vi "IMAQdx Calculate Frames per Second 1.vi"(0 "Session In":T1, 5 "Buffer Number":u32, 7 "Minimum Display Update Interval (ms)":u32=1000, 9 "Frames per Second Update Interval (ms)":u32=1000, 11 "error in (no error)":errorcluster, 12 "Reset Counters":bool) -> (3 "Update Display":bool, 4 "Session Out":T1, 6 "Acquired Frames per Second":dbl, 8 "Processed Frames per Second":dbl, 10 "Images Behind":i32, 14 "Images Missed":u32, 15 "error out":errorcluster)   [LabVIEW 2025, in "NI_Vision_Acquisition_Software.lvlib"]
doc: "Calculates the acquired and processing frame rate, the images behind, and images missed. This VI operates on a per-session basis, so it can be called with different IMAQdx camera sessions in parallel and it will return the calculated values for the session passed in."
uses:
  <vilib>/vision/driver/NI_Vision_Acquisition_Software.lvlib
  <vilib>/userDefined/High Color/IMAQdx.ctl
  <resource>/objmgr/imaqdx.rc
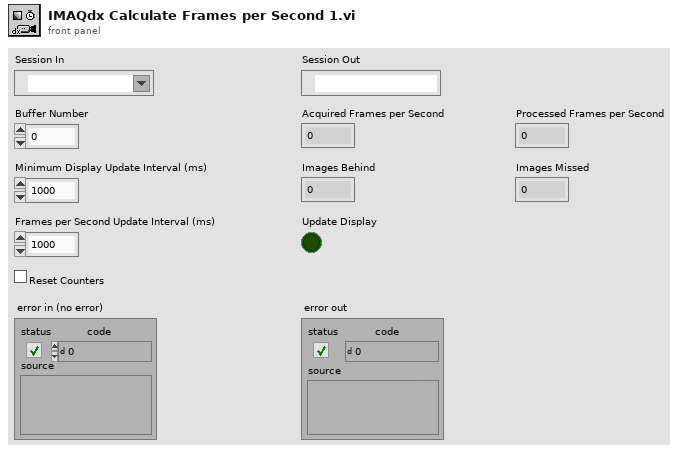
[diagram p1: front panel]
types:
  T1 = typedef "IMAQdx.ctl" = refnum<k21>
  T2 = cluster{"Last Display Timer Value":u32, "Last FPS Timer Value":u32, "Previous Buffer Number":i32, "Images Missed":u32, "Total Camera Frames":i32, "Last Acquired Frame Rate":dbl, "Last Processed Frame Rate":dbl, "Last Number of Processed Images":u32}
  T3 = cluster{"Last Display Timer Value":u32, "Last FPS Timer Value":u32, "Previous Buffer Number":i32, "Images Missed":u32, "Total Camera Frames":i32, "Last Acquired Frame Rate":dbl, "Last Processed Frame Rate":dbl, "Last Number of Processed Images":u32}[]
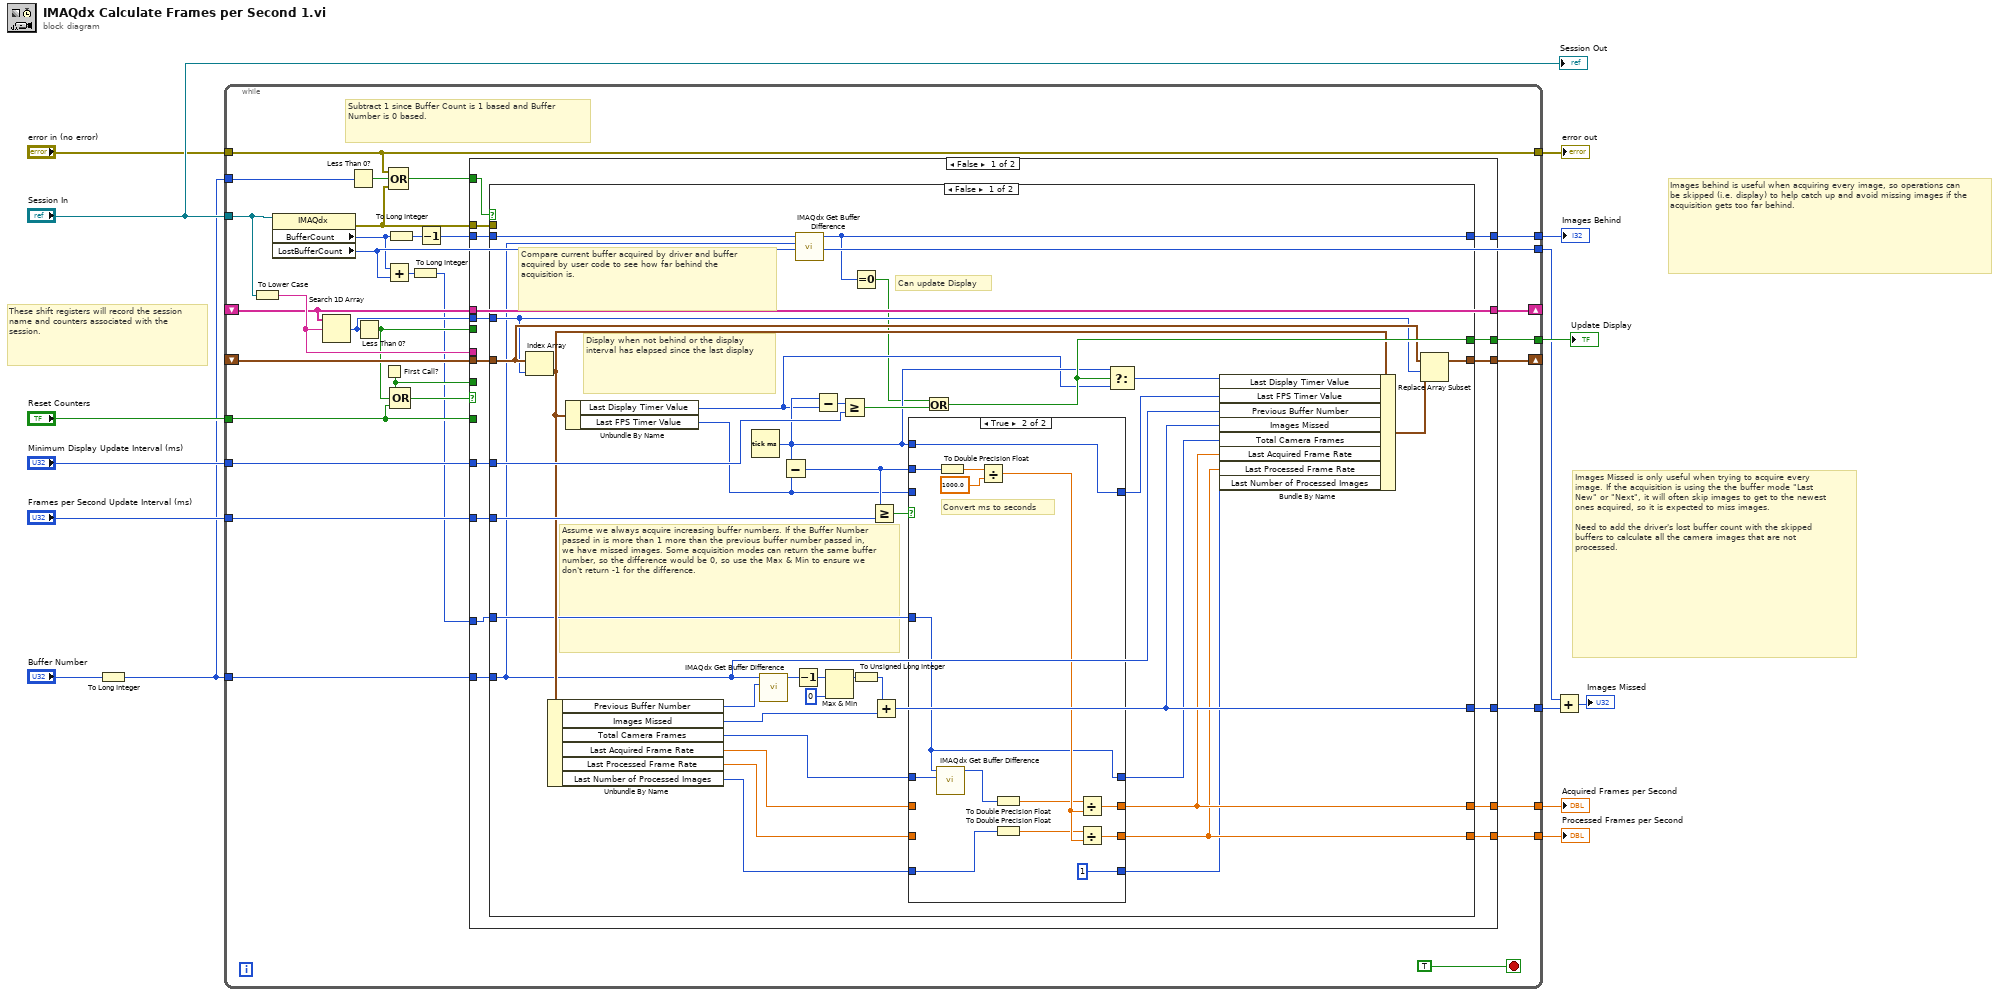
[diagram p0: block diagram]
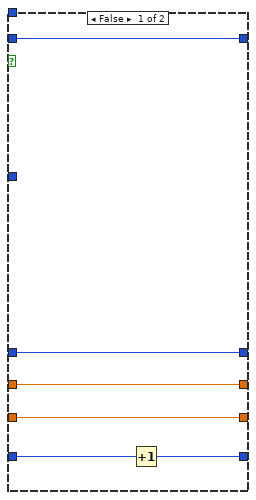
[diagram p2: hidden frame]
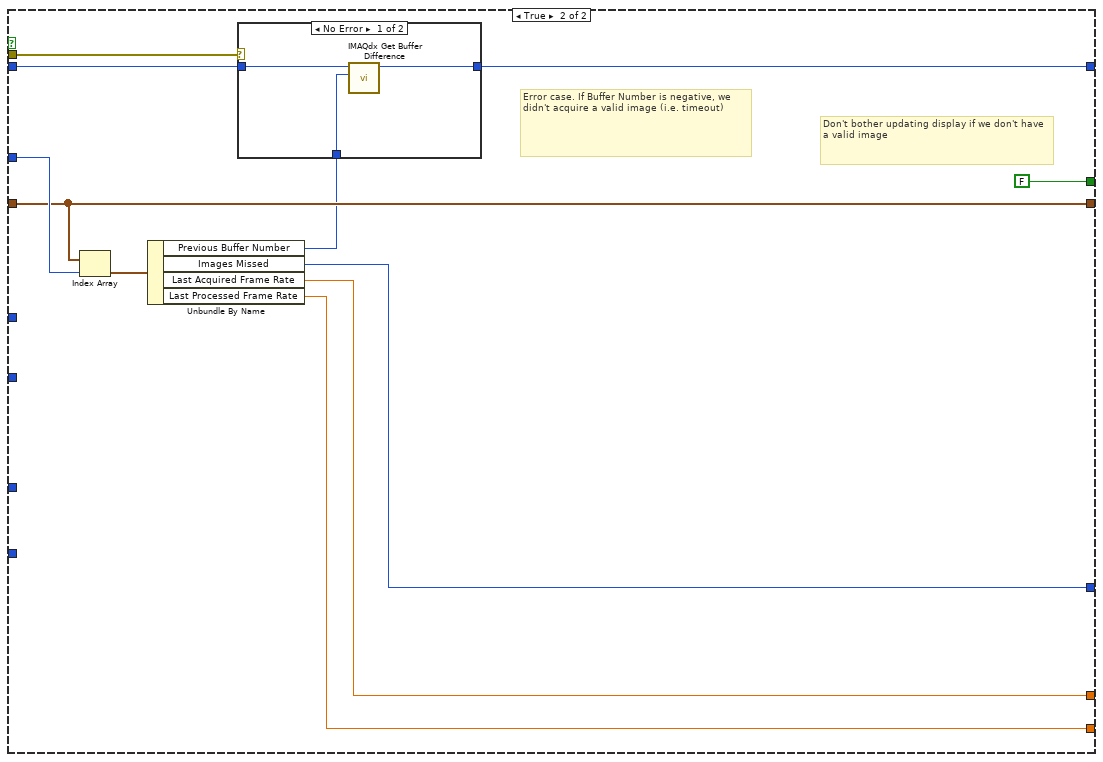
[diagram p3: hidden frame]
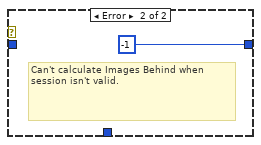
[diagram p4: hidden frame]
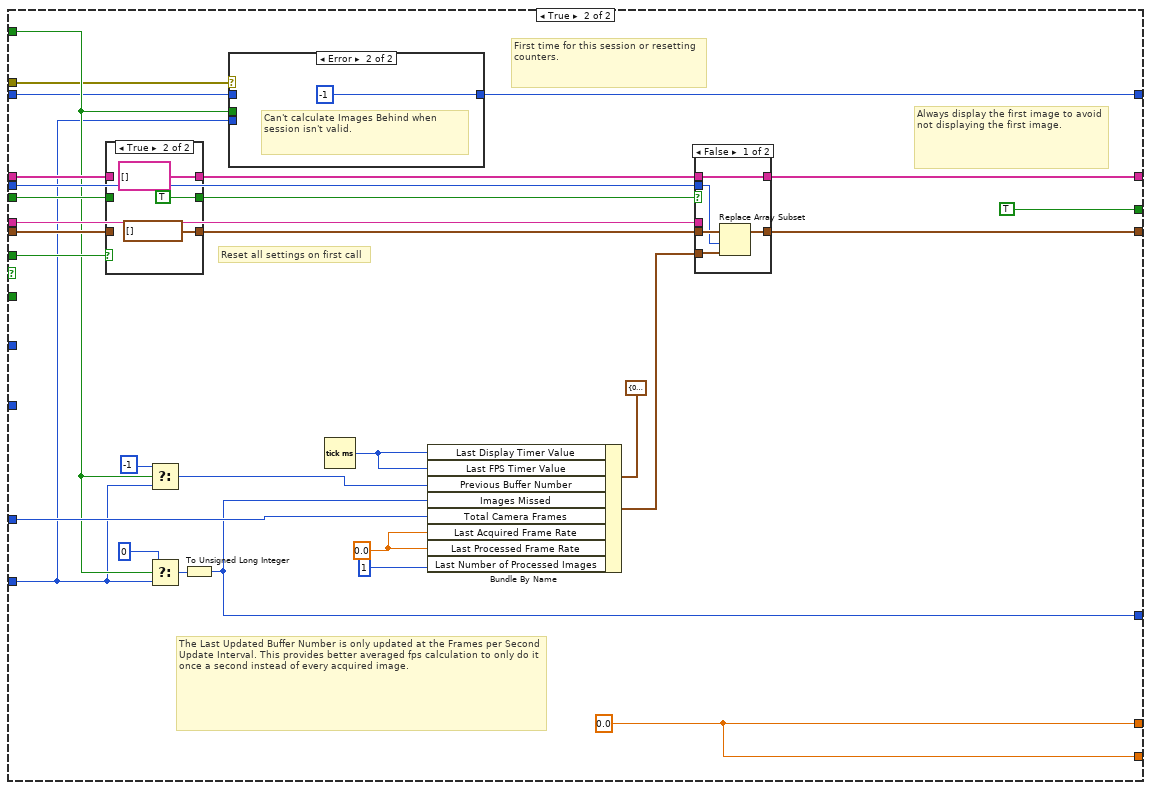
[diagram p5: hidden frame]
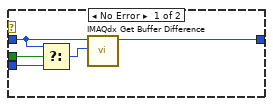
[diagram p6: hidden frame]
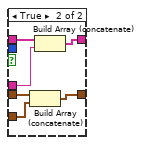
[diagram p8: hidden frame]
diagram:
  # "These shift registers will record the session name and counters associated with the session."
  # "Images behind is useful when acquiring every image, so operations can be skipped (i.e. display) to help catch up and avoid missing images if the acquisition gets too far behind."
  # "Images Missed is only useful when trying to acquire every image. If the acquisition is using the the buffer mode \"Last New\" or \"Next\", it will often skip images to get to the newest ones acquired, so it is expected to miss images. \n\nNeed to add the driver's lost buffer count with the skipped buffers to calculate all the camera images that are not processed."
  n1 = To Long Integer(number="Buffer Number") -> (32bit integer=w1:i32)
  n2 = while {
    tunnel: "Minimum Display Update Interval (ms)" -> [w45]
    tunnel: w1 -> [w44]
    tunnel: "Reset Counters" -> [w31]
    tunnel: "Session In" -> [w28]
    tunnel: [w19] -> w12
    tunnel: [w43] -> w11
    tunnel: "Frames per Second Update Interval (ms)" -> [w42]
    tunnel: [w24] -> w9
    tunnel: "error in (no error)" -> [w24]
    shift-right: [w41] -> _
    shift-left: _ -> [w40]
    tunnel: [w39] -> w5
    tunnel: [w38] -> w7
    tunnel: [w37] -> w6
    shift-right: [w34] -> _
    shift-left: _ -> [w33]
    tunnel: [w26] -> w4
    tunnel: w1 -> [w22]
    stop <- TRUE stop-if-true
    # "Subtract 1 since Buffer Count is 1 based and Buffer Number is 0 based."
    n3 = To Lower Case(string=w28) -> (all lower case string=w35:string)
    n4 = property class="IMAQdx"(reference=w28) -> (error out=w16:errorcluster, "BufferCount"=w20:u32, "LostBufferCount"=w26:u32)  [unwired: 1 in, 1 out]
    n5 = Search 1D Array(1D array=w33, element=w35) -> (index of element=w32:i32)  [unwired: 1 in]
    n6 = Less Than 0?(x=w22) -> (x < 0?=w25:bool)
    n7 = Less Than 0?(x=w32) -> (x < 0?=w30:bool)
    n8 = First Call?() -> (First Call?: T/F=w29:bool)
    n9 = Add(x=w20, y=w26) -> (x+y=w27:u32)
    n10 = To Long Integer(number=w20) -> (32bit integer=w18:i32)
    n11 = Compound Arithmetic op=OR(w24, w25, w16) -> (w23:bool)
    n12 = Compound Arithmetic op=OR(w29, w30, w31) -> (w36:bool)
    n13 = To Long Integer(number=w27) -> (32bit integer=w21:i32)
    n14 = Decrement(x=w18) -> (x-1=w17:i32)
    n15 = case shown="False" w36 {
      tunnel: [w57 w164] -> w38
      tunnel: w44 -> [w59 w139]
      tunnel: [w56 w164] -> w37
      tunnel: [w58 w141] -> w39
      tunnel: w31 -> [_ _]
      tunnel: [w61 TRUE] -> w43
      tunnel: w45 -> [w62 _]
      tunnel: w42 -> [w60 _]
      tunnel: [w54 w157] -> w41
      tunnel: w40 -> [w53 w153]
      tunnel: w30 -> [_ w148]
      tunnel: w33 -> [w55 w151]
      tunnel: w35 -> [_ w156]
      tunnel: [w55 w155] -> w34
      tunnel: w32 -> [w52 w149]
      tunnel: w29 -> [_ w154]
      tunnel: w21 -> [w51 w146]
      tunnel: w23 -> [w50 w140]
      tunnel: w17 -> [w49 w137]
      tunnel: [w48 w138] -> w19
      tunnel: w16 -> [w47 w136]
      frame False {
        n16 = case shown="False" w50 {
          tunnel: w62 -> [w98 _]
          tunnel: [w96 FALSE] -> w61
          tunnel: w60 -> [w89 _]
          tunnel: w59 -> [w63 _]
          tunnel: [w84 w127] -> w58
          tunnel: [w75 w129] -> w57
          tunnel: [w74 w128] -> w56
          tunnel: [w70 w130] -> w54
          tunnel: w53 -> [w69 w130]
          tunnel: w52 -> [w68 w131]
          tunnel: w51 -> [w67 _]
          tunnel: w49 -> [w65 w123]
          tunnel: [w64 w126] -> w48
          tunnel: w47 -> [_ w121]
          frame False {
            # "Compare current buffer acquired by driver and buffer acquired by user code to see how far behind the acquisition is."
            # "Can update Display"
            # "Display when not behind or the display interval has elapsed since the last display"
            # "Assume we always acquire increasing buffer numbers. If the Buffer Number passed in is more than 1 more than the previous buffer number passed in, we have missed images. Some acquisition modes can return the same buffer number, so the difference would be 0, so use the Max & Min to ensure we don't return -1 for the difference."
            n17 = Index Array(array=w69, index=w68) -> (element=w83:T2)
            n18 = Unbundle By Name(w83) -> ("Previous Buffer Number"=w82:i32, "Images Missed"=w80:u32, "Total Camera Frames"=w81:i32, "Last Acquired Frame Rate"=w78:dbl, "Last Processed Frame Rate"=w77:dbl, "Last Number of Processed Images"=w73:u32)
            n19 = Unbundle By Name(w83) -> ("Last Display Timer Value"=w88:u32, "Last FPS Timer Value"=w86:u32)
            n20 = Tick Count (ms)() -> (millisecond timer value=w95:u32)
            n21 = call <vilib>:"IMAQdx Get Buffer Difference.vi"("Previous Buffer Number"=w82, "Current BufferNumber"=w63) -> ("Buffer Difference"=w93:i32)  [unwired: 9 in]
            n22 = Subtract(x=w95, y=w86) -> (x-y=w99:u32)
            n23 = Decrement(x=w93) -> (x-1=w92:i32)
            n24 = call <vilib>:"IMAQdx Get Buffer Difference.vi"("Previous Buffer Number"=w63, "Current BufferNumber"=w65) -> ("Buffer Difference"=w64:i32)  [unwired: 9 in]
            n25 = Subtract(x=w95, y=w88) -> (x-y=w94:u32)
            n26 = Max & Min(x=w92, y=0) -> (max(x,y)=w90:i32)  [unwired: 1 out]
            n27 = Greater Or Equal?(x=w94, y=w98) -> (x >= y?=w97:bool)
            n28 = Equal To 0?(x=w64) -> (x = 0?=w66:bool)
            n29 = To Unsigned Long Integer(number=w90) -> (unsigned 32bit integer=w79:u32)
            n30 = Greater Or Equal?(x=w99, y=w89) -> (x >= y?=w100:bool)
            n31 = Add(x=w79, y=w80) -> (x+y=w84:u32)
            n32 = case shown="True" w100 {
              tunnel: w86 -> [w106 _]
              tunnel: [w106 w120] -> w85
              tunnel: w81 -> [w104 w115]
              tunnel: [w104 w108] -> w76
              tunnel: w95 -> [_ w120]
              tunnel: w99 -> [_ w117]
              tunnel: [w105 w119] -> w75
              tunnel: w78 -> [w105 _]
              tunnel: w67 -> [_ w108]
              tunnel: w73 -> [w103 w109]
              tunnel: [w102 u32 1] -> w72
              tunnel: [w101 w116] -> w74
              tunnel: w77 -> [w101 _]
              frame False {
                n33 = Increment(x=w103) -> (x+1=w102:u32)
              }
              frame True {
                # "Convert ms to seconds"
                n34 = call <vilib>:"IMAQdx Get Buffer Difference.vi"("Previous Buffer Number"=w115, "Current BufferNumber"=w108) -> ("Buffer Difference"=w114:i32)  [unwired: 9 in]
                n35 = To Double Precision Float(number=w117) -> (double precision float=w113:dbl)
                n36 = Divide(x=w113, y=1000.0) -> (x/y=w111:dbl)
                n37 = To Double Precision Float(number=w114) -> (double precision float=w110:dbl)
                n38 = To Double Precision Float(number=w109) -> (double precision float=w107:dbl)
                n39 = Divide(x=w110, y=w111) -> (x/y=w119:dbl)
                n40 = Divide(x=w107, y=w111) -> (x/y=w116:dbl)
              }
            }
            n41 = Or(x=w66, y=w97) -> (x .or. y?=w96:bool)
            n42 = Select(t=w95, s=w96, f=w88) -> (s? t:f=w87:u32)
            n43 = Bundle By Name(cluster=w83, "Last Display Timer Value"=w87, "Last FPS Timer Value"=w85, "Previous Buffer Number"=w63, "Images Missed"=w84, "Total Camera Frames"=w76, "Last Acquired Frame Rate"=w75, "Last Processed Frame Rate"=w74, "Last Number of Processed Images"=w72) -> (w71:T2)
            n44 = Replace Array Subset(array=w69, new element=w71, index=w68) -> (w70:T3)
          }
          frame True {
            # "Don't bother updating display if we don't have a valid image"
            # "Error case. If Buffer Number is negative, we didn't acquire a valid image (i.e. timeout)"
            n45 = Index Array(array=w130, index=w131) -> (element=w125:T2)
            n46 = Unbundle By Name(w125) -> ("Previous Buffer Number"=w124:i32, "Images Missed"=w127:u32, "Last Acquired Frame Rate"=w129:dbl, "Last Processed Frame Rate"=w128:dbl)
            n47 = case shown="No Error" w121 {
              tunnel: [w134 -1 ("Buffer Difference")] -> w126
              tunnel: w124 -> [w133 _]
              tunnel: w123 -> [w132 _]
              frame No Error {
                n48 = call <vilib>:"IMAQdx Get Buffer Difference.vi"("Previous Buffer Number"=w133, "Current BufferNumber"=w132) -> ("Buffer Difference"=w134:i32)  [unwired: 9 in]
              }
              frame Error {
                # "Can't calculate Images Behind when session isn't valid."
              }
            }
          }
        }
      }
      frame True {
        w161 = 0.0
        w164 = 0.0
        # "First time for this session or resetting counters."
        # "Reset all settings on first call"
        # "The Last Updated Buffer Number is only updated at the Frames per Second Update Interval. This provides better averaged fps calculation to only do it once a second instead of every acquired image."
        # "Always display the first image to avoid not displaying the first image."
        n49 = case shown="True" w154 {
          tunnel: w153 -> [w173 _]
          tunnel: [w173 T3 []] -> w152
          tunnel: w151 -> [w172 _]
          tunnel: [w172 string[] []] -> w150
          tunnel: w148 -> [w171 _]
          tunnel: [w171 TRUE] -> w147
          frame False {
          }
          frame True {
          }
        }
        n50 = Select(t=-1, s=w140, f=w139) -> (s? t:f=w143:i32)
        n51 = Select(t=0, s=w140, f=w139) -> (s? t:f=w144:i32)
        n52 = To Unsigned Long Integer(number=w144) -> (unsigned 32bit integer=w141:u32)
        n53 = case shown="Error" w136 {
          tunnel: w140 -> [w169 _]
          tunnel: w139 -> [w168 _]
          tunnel: [w166 -1 ("Buffer Difference")] -> w138
          tunnel: w137 -> [w165 _]
          frame No Error {
            n54 = Select(t=w165, s=w169, f=w168) -> (s? t:f=w167:i32)
            n55 = call <vilib>:"IMAQdx Get Buffer Difference.vi"("Previous Buffer Number"=w167, "Current BufferNumber"=w165) -> ("Buffer Difference"=w166:i32)  [unwired: 9 in]
          }
          frame Error {
            # "Can't calculate Images Behind when session isn't valid."
          }
        }
        n56 = Tick Count (ms)() -> (millisecond timer value=w162:u32)
        n57 = Bundle By Name(cluster=T2 {"Last Display Timer Value"=0, "Last FPS Timer Value"=0, "Previous Buffer Number"=0, "Images Missed"=0, "Total Camera Frames"=0, "Last Acquired Frame Rate"=0.0, "Last Processed Frame Rate"=0.0, "Last Number of Processed Images"=0} ("output cluster"), "Last Display Timer Value"=w162, "Last FPS Timer Value"=w162, "Previous Buffer Number"=w143, "Images Missed"=w141, "Total Camera Frames"=w146, "Last Acquired Frame Rate"=w161, "Last Processed Frame Rate"=w161, "Last Number of Processed Images"=u32 1) -> (w158:T2)
        n58 = case shown="False" w147 {
          tunnel: w158 -> [w178 w187]
          tunnel: [w179 w186] -> w157
          tunnel: w152 -> [w180 w185]
          tunnel: w156 -> [_ w184]
          tunnel: [w181 w183] -> w155
          tunnel: w150 -> [w181 w182]
          tunnel: w149 -> [w177 _]
          frame False {
            n59 = Replace Array Subset(array=w180, new element=w178, index=w177) -> (w179:T3)
          }
          frame True {
            n60 = Build Array (concatenate)(w185, w187) -> (w186:T3)
            n61 = Build Array (concatenate)(w182, w184) -> (w183:string[])
          }
        }
      }
    }
  }
  "Acquired Frames per Second" <- w7
  "Processed Frames per Second" <- w6
  "Images Behind" <- w12
  "Update Display" <- w11
  "error out" <- w9
  n62 = Add(x=w4, y=w5) -> (x+y=→"Images Missed":u32)
  "Session Out" <- "Session In"
